vi "DatabaseControllerGFV.vi"(8 "error in (no error)":errorcluster, 10 "Enum":T1, 11 "Data in":variant) -> (0 "error out":errorcluster, 3 "Data Out":variant)   [LabVIEW 2017]
doc: "Use this template to build a VI to use as a subVI."
uses:
  DatabaseContollerGFVenum.ctl
  <vilib>/addons/Database/Connection.llb/Conn ObjectReference.ctl
  <vilib>/addons/Database/Connection.llb/DB Tools Open Connec (Path).vi
  <vilib>/addons/Database/Connection.llb/Conn Execute.vi
  <vilib>/addons/Database/Recordset.llb/Rec Fetch String Data (R).vi
  <vilib>/addons/Database/Recordset.llb/Rec Move To Next Record (R).vi
  <vilib>/addons/Database/Recordset.llb/Rec Destroy - Connection.vi
  <vilib>/addons/Database/NI_Database_API.lvlib
panel:
  out "Images":string[](array[string])
  out "Names":string[](array[string])
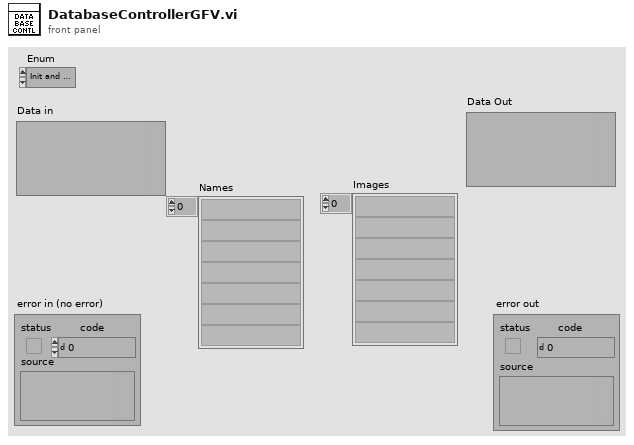
[diagram p1: front panel]
types:
  T1 = typedef "DatabaseContollerGFVenum.ctl" = enum16{"Init and Open Database!", "Close Database!", "Get Users!"}
  T2 = typedef "NI_Database_API.lvlib/Conn ObjectReference.ctl" = refnum<k1>
  T3 = typedef "NI_Database_API.lvlib/Rec ObjectReference.ctl" = refnum<k1>
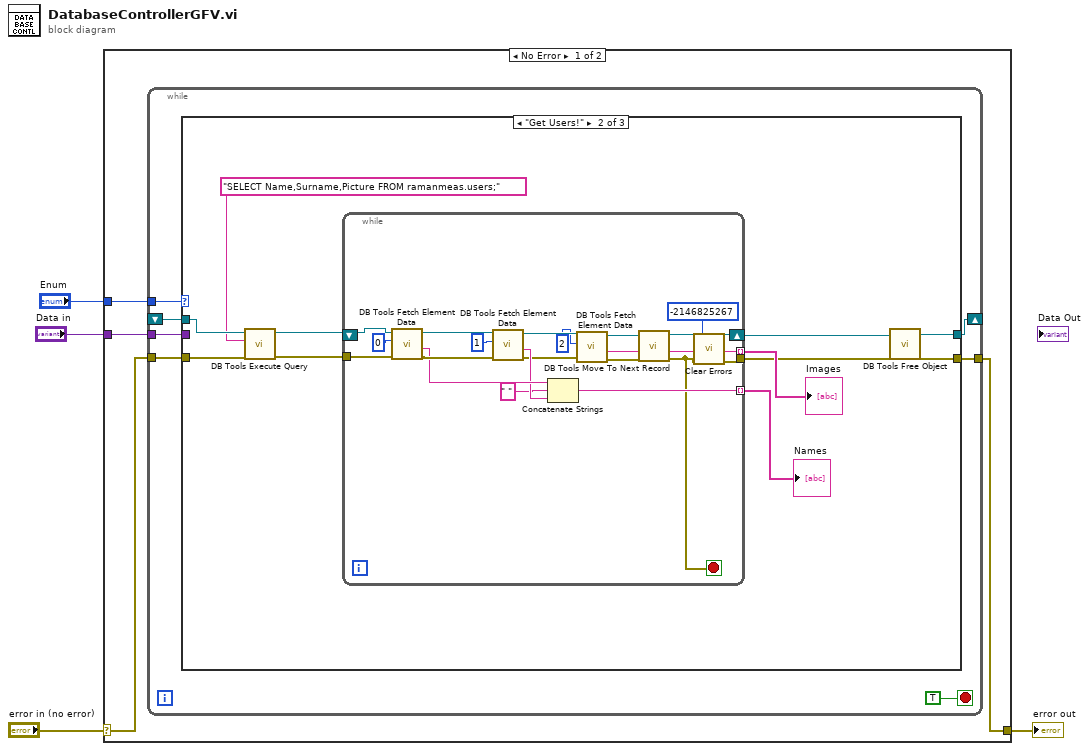
[diagram p0: block diagram]
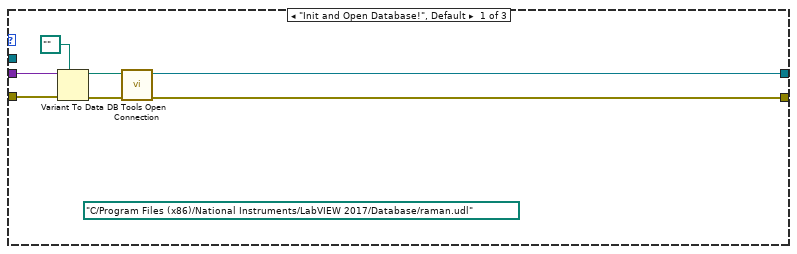
[diagram p2: hidden frame]
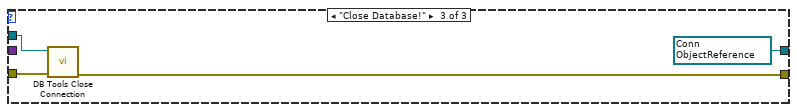
[diagram p3: hidden frame]
diagram:
  n1 = case shown="No Error" "error in (no error)" {
    selector: "error in (no error)" -> [w6 w58]
    tunnel: [w5 w58] -> w3
    tunnel: "Enum" -> [w8 _]
    tunnel: "Data in" -> [w7 _]
    frame No Error {
      n2 = while {
        tunnel: w8 -> [w14]
        tunnel: w7 -> [w13]
        tunnel: w6 -> [w12]
        tunnel: [w11] -> w5
        shift-right: [w10] -> _
        shift-left: _ -> [w9]
        stop <- TRUE stop-if-true
        n3 = case shown="\"Get Users!\"" w14 {
          tunnel: w13 -> [w22 _ _]
          tunnel: w12 -> [w21 w33 w57]
          tunnel: [w18 w29 w55] -> w11
          tunnel: [w16 w28 w54] -> w10
          tunnel: w9 -> [_ w32 w56]
          frame "Init and Open Database!", Default {
            (unwired) path "C:/Program Files (x86)/National Instruments/LabVIEW 2017/Database/raman.udl" ("connection information")
            n4 = Variant To Data(error in=w21, type=path "" ("connection information"), Variant=w22) -> (data=w17:path, error out=w19:errorcluster)
            n5 = call-poly <vilib>:"DB Tools Open Connection.vi"("error in (no error)"=w19, "connection information"=w17) -> ("error out"=w18:errorcluster, "connection reference"=w16:T2)  [unwired: 6 in]
          }
          frame "Get Users!" {
            n6 = call-poly <vilib>:"DB Tools Execute Query.vi"("error in (no error)"=w33, "SQL query"="SELECT Name,Surname,Picture FROM ramanmeas.users;", "connection reference"=w32) -> ("error out"=w31:errorcluster, "recordset reference"=w30:T3)  [unwired: 5 in]
            n7 = while {
              tunnel: w31 -> [w53]
              tunnel: [w44] -> w26 mode=indexing
              shift-right: [w38] -> w24
              shift-left: w30 -> [w52]
              tunnel: [w41] -> w25 mode=indexing
              tunnel: [w34] -> w23
              stop <- w35 stop-if-true
              n8 = call-poly <vilib>:"DB Tools Fetch Element Data.vi"("error in (no error)"=w53, "column index"=0, "recordset reference"=w52) -> ("error out"=w48:errorcluster, "data"=w47:string, "recordset reference out"=w49:T3)  [unwired: 4 in]
              n9 = call-poly <vilib>:"DB Tools Fetch Element Data.vi"("error in (no error)"=w48, "column index"=1, "recordset reference"=w49) -> ("error out"=w43:errorcluster, "data"=w46:string, "recordset reference out"=w42:T3)  [unwired: 4 in]
              n10 = Concatenate Strings(w47, " " ("string"), w46) -> (w44:string)
              n11 = call-poly <vilib>:"DB Tools Fetch Element Data.vi"("error in (no error)"=w43, "column index"=2, "recordset reference"=w42) -> ("error out"=w40:errorcluster, "data"=w41:string, "recordset reference out"=w39:T3)  [unwired: 4 in]
              n12 = call-poly <vilib>:"DB Tools Move To Next Record.vi"("error in (no error)"=w40, "recordset reference"=w39) -> ("error out"=w35:errorcluster, "recordset reference out"=w38:T3)  [unwired: 8 in]
              n13 = call <vilib>:"Clear Errors.vi"("error in (no error)"=w35, "specific error code to clear (0: all)"=-2146825267) -> ("error out"=w34:errorcluster)  [unwired: 4 in, 1 out]
            }
            "Names" <- w26
            "Images" <- w25
            n14 = call-poly <vilib>:"DB Tools Free Object.vi"("error in (no error)"=w23, "recordset reference"=w24) -> ("error out"=w29:errorcluster, "connection reference"=w28:T2)  [unwired: 8 in]
          }
          frame "Close Database!" {
            w54 = T2 refnum items=["Connection"] ("connection reference")
            n15 = call <vilib>:"DB Tools Close Connection.vi"("error in (no error)"=w57, "connection reference"=w56) -> ("error out"=w55:errorcluster)  [unwired: 5 in]
          }
        }
      }
    }
    frame Error {
    }
  }
  "error out" <- w3
